vi "RGB TO RY.vi"(11 "Array":u8[](array[numeric])) -> (3 "Mean Value of Ry":dbl format="%0.2f")   [LabVIEW 2020]
uses:
  <vilib>/Analysis/baseanly.llb/Mean (DBL).vi
  <vilib>/Analysis/NI_AALBase.lvlib
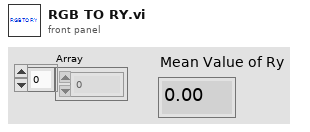
[diagram p1: front panel]
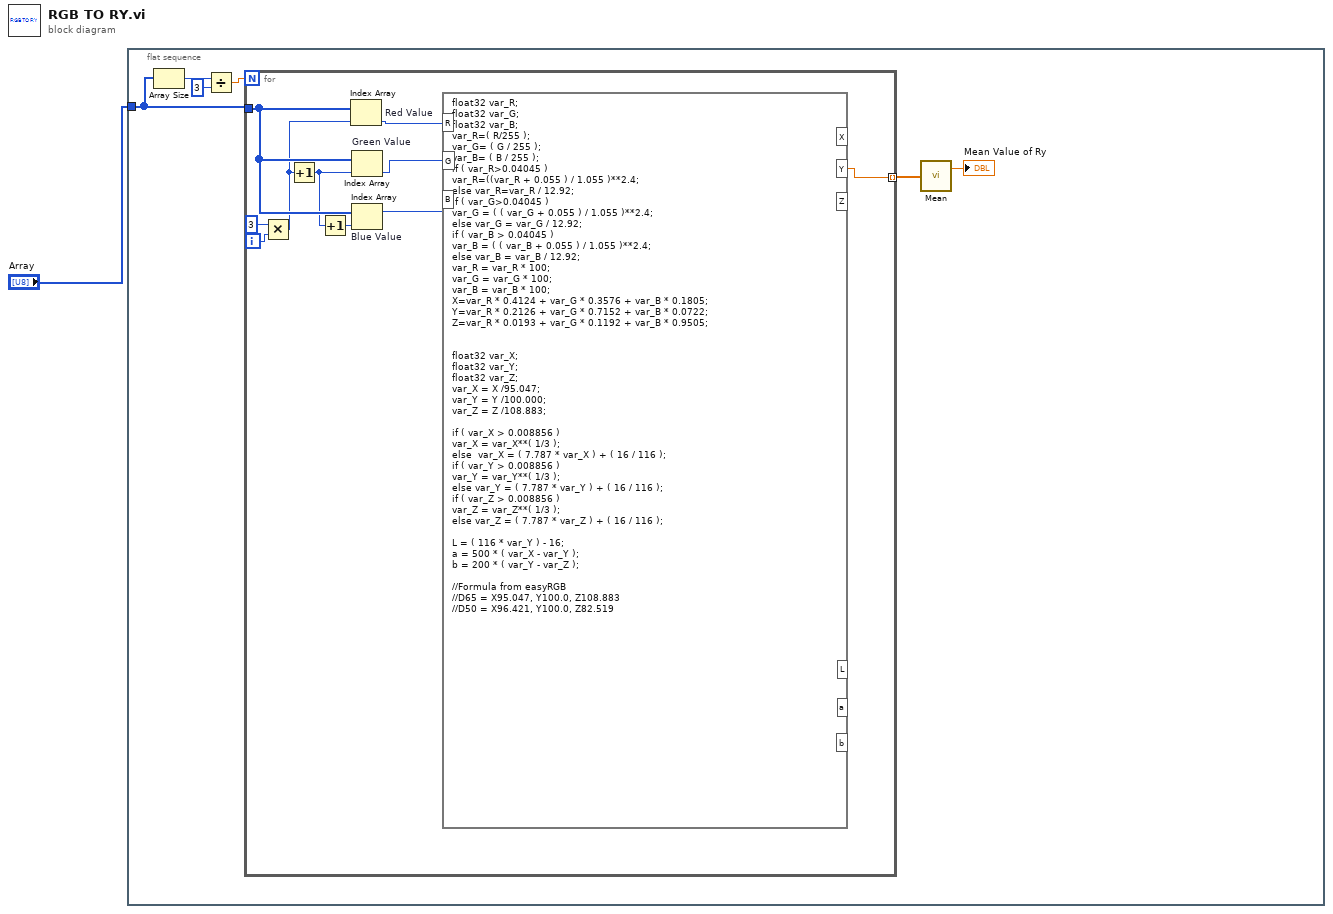
[diagram p0: block diagram]
diagram:
  n1 = flat-sequence {
    tunnel: "Array" -> [w5]
    frame #0 {
      n2 = Array Size(array=w5) -> (size(s)=w6:i32)
      n3 = Divide(x=w6, y=3 ("x")) -> (x/y=w4:dbl)
      n4 = for {
        N: w4 -> [_]
        tunnel: w5 -> [w15]
        tunnel: [w8] -> w3 mode=indexing
        i -> [w17]
        n5 = Multiply(x=3, y=w17) -> (x*y=w13:i32)
        n6 = Increment(x=w13) -> (x+1=w14:i32)
        n7 = Increment(x=w14) -> (x+1=w12:i32)
        n8 = Index Array "Red Value"(array=w15, index=w13) -> (element=w11:u8)
        n9 = Index Array "Green Value"(array=w15, index=w14) -> (element=w10:u8)
        n10 = Index Array "Blue Value"(array=w15, index=w12) -> (element=w9:u8)
        n11 = formula code="float32 var_R;\nfloat32 var_G;\nfloat32 var_B;\nvar_R=( R/255 );\nvar_G= ( G / 255 );\nvar_B= ( B / 255 );\nif ( var_R>0.04045 )\nvar_R=((var_R + 0.055 ) / 1.055 )**2.4;\nelse var_R=var_R / 12.92;\nif ( var_G>0.04045 ) \nvar_G = ( ( var_G + 0.055 ) / 1.055 )**2.4;\nelse var_G = var_G / 12.92;\nif ( var_B > 0.04045 ) \nvar_B = ( ( var_B + 0.055 ) / 1.055 )**2.4;\nelse var_B = var_B / 12.92;\nvar_R = var_R * 100;\nvar_G = var_G * 100;\nvar_B = var_B * 100;\nX=var_R * 0.4124 + var_G * 0.3576 + var_B * 0.1805;\nY=var_R * 0.2126 + var_G * 0.7152 + var_B * 0.0722;\nZ=var_R * 0.0193 + var_G * 0.1192 + var_B * 0.9505;\n\n\nfloat32 var_X;\nfloat32 var_Y;\nfloat32 var_Z;\nvar_X = X /95.047;\nvar_Y = Y /100.000;\nvar_Z = Z /108.883;\n\nif ( var_X > 0.008856 ) \nvar_X = var_X**( 1/3 );\nelse  var_X = ( 7.787 * var_X ) + ( 16 / 116 );\nif ( var_Y > 0.008856 ) \nvar_Y = var_Y**( 1/3 );\nelse var_Y = ( 7.787 * var_Y ) + ( 16 / 116 );\nif ( var_Z > 0.008856 ) \nvar_Z = var_Z**( 1/3 );\nelse var_Z = ( 7.787 * var_Z ) + ( 16 / 116 );\n\nL = ( 116 * var_Y ) - 16;\na = 500 * ( var_X - var_Y );\nb = 200 * ( var_Y - var_Z );\n\n//Formula from easyRGB\n//D65 = X95.047, Y100.0, Z108.883\n//D50 = X96.421, Y100.0, Z82.519"("R"=w11, "G"=w10, "B"=w9) -> ("Y"=w8:dbl)  [unwired: 5 out]
      }
      n12 = call-poly <vilib>:"Mean.vi"("X"=w3) -> ("mean"=→"Mean Value of Ry":dbl)  [unwired: 1 out]
    }
  }
